vi "UpdateVisibleData.vi"(7 "Templates tree":refnum<vi>, 8 "error in (no error)":errorcluster, 9 "Tag":string, 10 "Keyword":string, 11 "FakedArray in":refnum<class "FakedArray.lvclass">) -> (0 "error out":errorcluster, 3 "FakedArray out":refnum<class "FakedArray.lvclass">)   [LabVIEW 2020, in "FakedArray.lvclass"]
uses:
  FakedArray.lvclass
  FakedArray.lvclass/FakedArray.ctl
  vi.lib/LabVIEW Icon API/lv_icon/Classes/Layer/Layer.lvclass
  vi.lib/LabVIEW Icon API/LabVIEW Icon API.lvlib
  Icon Library/Glyph.lvclass
  vi.lib/LabVIEW Icon API/lv_icon/Controls/Graphic.ctl
panel:
  in  "?":T1
  in  "?":T1[](array[typedef])=[{"Rectangle"={"left"=0, "top"=0, "right"=0, "bottom"=0}, "Path"=path "", "Image"=bytes[0], "Filter"="", "FileName"=""}]
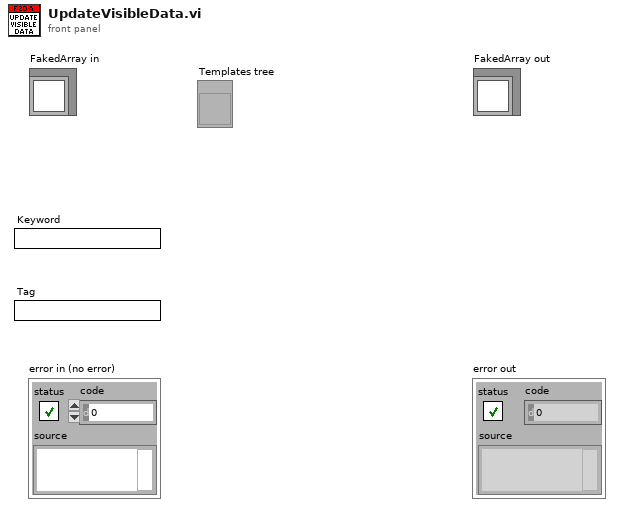
[diagram p1: front panel]
types:
  T1 = typedef "Graphic.ctl" = cluster{"Rectangle":cluster{"left":i16, "top":i16, "right":i16, "bottom":i16}, "Path":path, "Image":picture, "Filter":string, "FileName":string}
  T2 = typedef "ToMoreSpecific_Faked2DArray.ctl" = enum16{"Framework Templates", "Layer List"}
  T3 = typedef "IEColor.ctl" = u32
  T4 = typedef "Path&Icon.ctl" = cluster{"Rectangle":cluster{"left":i16, "top":i16, "right":i16, "bottom":i16}, "Path":path, "Image":picture, "Filter":string, "FileName":string}
  T5 = cluster{"Rectangle":cluster{"left":bool, "top":bool, "right":bool, "bottom":bool}, "Path":bool, "Image":bool, "Filter":bool, "FileName":bool}
  T6 = typedef "Layer.ctl" = cluster{"LayerIcon":picture, "LayerName":string, "Opacity":u8, "Visibility?":bool}
  T7 = typedef "LVPoint32TypeDef.ctl" = cluster{"Horizontal":i32, "Vertical":i32}
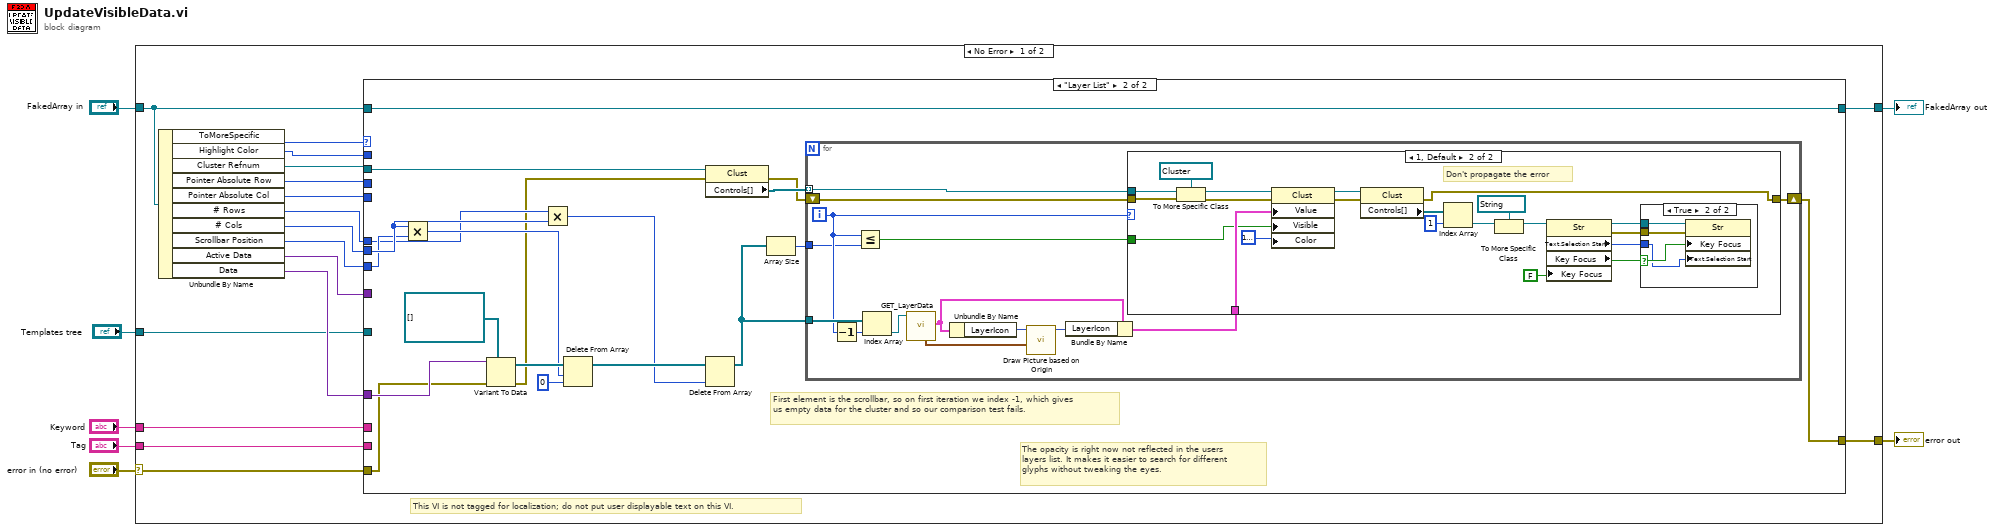
[diagram p0: block diagram]
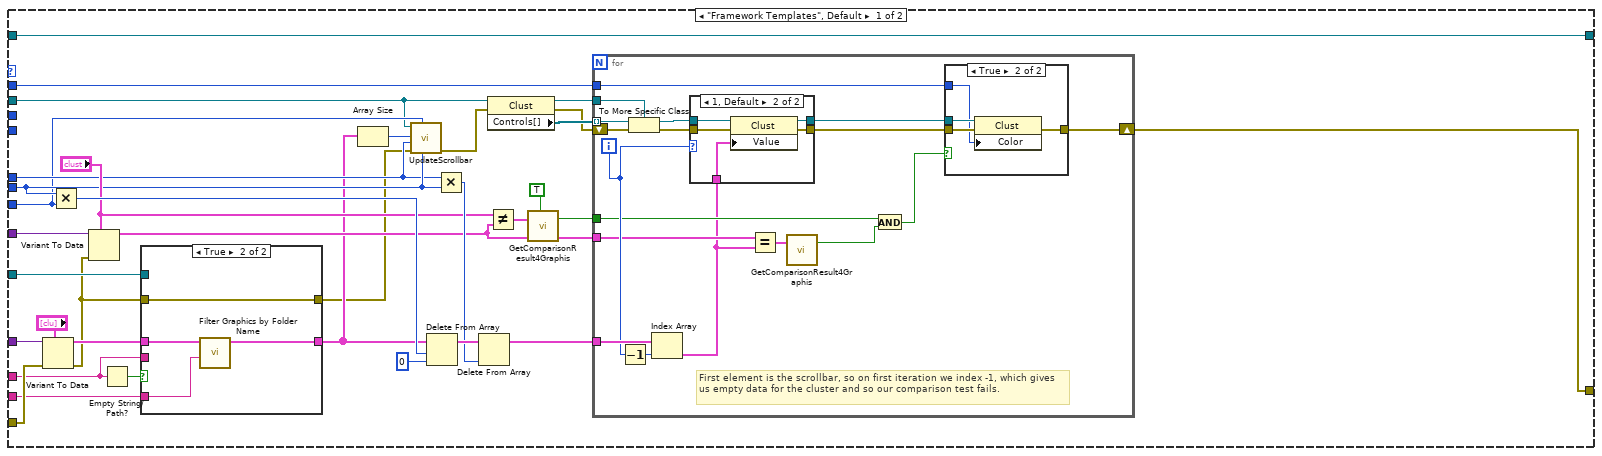
[diagram p2: hidden frame]
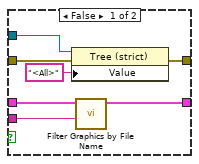
[diagram p3: hidden frame]
diagram:
  n1 = case shown="No Error" "error in (no error)" {
    selector: "error in (no error)" -> [w22 w159]
    tunnel: [w18 w159] -> w6
    tunnel: [w17 w158] -> w4
    tunnel: "FakedArray in" -> [w24 w158]
    tunnel: "Keyword" -> [w14 _]
    tunnel: "Tag" -> [w10 _]
    tunnel: "Templates tree" -> [w8 _]
    frame No Error {
      # "This VI is not tagged for localization; do not put user displayable text on this VI."
      n2 = Unbundle By Name(w24) -> ("ToMoreSpecific"=w9:T2, "Highlight Color"=w11:T3, "Cluster Refnum"=w19:refnum<vi>, "Pointer Absolute Row"=w16:i32, "Pointer Absolute Col"=w15:i32, "# Rows"=w20:i32, "# Cols"=w21:i32, "Scrollbar Position"=w23:i32, "Active Data"=w12:variant, "Data"=w13:variant)
      n3 = case shown="\"Layer List\"" w9 {
        tunnel: w24 -> [w47 w112]
        tunnel: w23 -> [w30 w106]
        tunnel: w13 -> [w58 w117]
        tunnel: w22 -> [w57 w116]
        tunnel: w21 -> [w32 w107]
        tunnel: w20 -> [w31 w102]
        tunnel: w19 -> [w29 w111]
        tunnel: [w48 w113] -> w18
        tunnel: [w47 w112] -> w17
        tunnel: w16 -> [_ _]
        tunnel: w15 -> [_ _]
        tunnel: w14 -> [w43 _]
        tunnel: w12 -> [w42 _]
        tunnel: w11 -> [w37 _]
        tunnel: w10 -> [w35 _]
        tunnel: w8 -> [w34 _]
        frame "Framework Templates", Default {
          n4 = Variant To Data(error in=w57, type="?", Variant=w58) -> (data=w45:T1[], error out=w33:errorcluster)
          n5 = Multiply(x=w32, y=w30) -> (x*y=w55:i32)
          n6 = Variant To Data(error in=w33, type="?", Variant=w42) -> (data=w40:T1)  [unwired: 1 out]
          n7 = Empty String/Path?(string/path=w43) -> (empty?=w44:bool)
          n8 = case shown="True" w44 {
            tunnel: w45 -> [w65 w69]
            tunnel: w43 -> [w64 _]
            tunnel: [w63 w68] -> w28
            tunnel: w35 -> [_ w67]
            tunnel: w33 -> [w60 w66]
            tunnel: [w62 w66] -> w26
            tunnel: w34 -> [w61 _]
            frame False {
              n9 = property class="Tree (strict)"(reference=w61, error in=w60, "Value"="<All>") -> (error out=w62:errorcluster)  [unwired: 1 out]
              n10 = call "Filter Graphics by File Name.vi"("Keyword"=w64, "Icon Templates in"=w65) -> ("Icon Templates out"=w63:T4[])  [unwired: 9 out]
            }
            frame True {
              n11 = call "Filter Graphics by Folder Name.vi"("Tag"=w67, "Glyphs [] in"=w69) -> ("Filtered Glyphs []"=w68:T1[])  [unwired: 9 out]
            }
          }
          n12 = Array Size(array=w28) -> (size(s)=w27:i32)
          n13 = call "UpdateScrollbar.vi"("# Cols"=w32, "Value Scrollbar"=w30, "error in"=w26, "#Rows"=w31, "# Elements"=w27, "Cluster Refnum"=w29) -> ("error out"=w25:errorcluster)  [unwired: 5 out]
          n14 = Delete From Array(array=w28, length=w55, index=0) -> (array with subset deleted=w53:T1[])  [unwired: 1 out]
          n15 = Multiply(x=w31, y=w32) -> (x*y=w52:i32)
          n16 = Delete From Array(array=w53, index=w52) -> (array with subset deleted=w49:T1[])  [unwired: 1 in, 1 out]
          n17 = property class="Clust"(reference=w29, error in=w25) -> (reference out=w46:refnum<vi>, error out=w50:errorcluster, "Controls[]"=w51:refnum<vi>[])
          n18 = Not Equal?(x="?", y=w40) -> (x != y?=w39:T5)
          n19 = call "GetComparisonResult4Graphis.vi"("Comparison In"=w39, "AND vs OR"=TRUE) -> ("True?"=w38:bool)  [unwired: 17 out]
          n20 = for {
            tunnel: w51 -> [w74] mode=indexing
            shift-right: [w76] -> w48
            shift-left: w50 -> [w73]
            tunnel: w49 -> [w87]
            tunnel: w46 -> [w75]
            tunnel: w40 -> [w84]
            tunnel: w38 -> [w82]
            tunnel: w37 -> [w77]
            i -> [w85]
            # "First element is the scrollbar, so on first iteration we index -1, which gives us empty data for the cluster and so our comparison test fails."
            n21 = Decrement(x=w85) -> (x-1=w86:i32)
            n22 = To More Specific Class(target class=w75, reference=w74, error in=w73) -> (specific class reference=w71:refnum<vi>, error out=w72:errorcluster)
            n23 = Index Array(array=w87, index=w86) -> (element=w70:T1)
            n24 = case shown="1, Default" w85 {
              tunnel: w71 -> [w93 w98]
              tunnel: [_ w97] -> w83
              tunnel: w70 -> [_ w96]
              tunnel: [w93 w95] -> w78
              tunnel: w72 -> [_ w94]
              frame 0 {
                # "Do not propagate\nerror! This is the\nscrollbar."
              }
              frame 1, Default {
                n25 = property class="Clust"(reference=w98, error in=w94, "Value"=w96) -> (reference out=w95:refnum<vi>, error out=w97:errorcluster)
              }
            }
            n26 = Equal?(x=w84, y=w70) -> (x = y?=w81:T5)
            n27 = call "GetComparisonResult4Graphis.vi"("Comparison In"=w81) -> ("True?"=w80:bool)  [unwired: 1 in, 17 out]
            n28 = And(x=w82, y=w80) -> (x .and. y?=w79:bool)
            n29 = case shown="True" w79 {
              tunnel: w83 -> [w88 w92]
              tunnel: w78 -> [_ w91]
              tunnel: w77 -> [_ w89]
              tunnel: [w88 w90] -> w76
              frame False {
              }
              frame True {
                n30 = property class="Clust"(reference=w91, error in=w92, "Color"=w89) -> (error out=w90:errorcluster)  [unwired: 1 out]
              }
            }
          }
        }
        frame "Layer List" {
          # "The opacity is right now not reflected in the users\nlayers list. It makes it easier to search for different\nglyphs without tweaking the eyes."
          # "First element is the scrollbar, so on first iteration we index -1, which gives us empty data for the cluster and so our comparison test fails."
          n31 = Multiply(x=w107, y=w106) -> (x*y=w103:i32)
          n32 = Variant To Data(error in=w116, type=refnum<class "Layer.lvclass">[] [] ("All Layers"), Variant=w117) -> (data=w104:refnum<class "Layer.lvclass">[], error out=w99:errorcluster)
          n33 = Multiply(x=w102, y=w107) -> (x*y=w100:i32)
          n34 = Delete From Array(array=w104, length=w103, index=0) -> (array with subset deleted=w108:refnum<class "Layer.lvclass">[])  [unwired: 1 out]
          n35 = property class="Clust"(reference=w111, error in=w99) -> (error out=w114:errorcluster, "Controls[]"=w115:refnum<vi>[])  [unwired: 1 out]
          n36 = Delete From Array(array=w108, index=w100) -> (array with subset deleted=w105:refnum<class "Layer.lvclass">[])  [unwired: 1 in, 1 out]
          n37 = Array Size(array=w105) -> (size(s)=w109:i32)
          n38 = for {
            tunnel: w115 -> [w131] mode=indexing
            shift-right: [w129] -> w113
            shift-left: w114 -> [w130]
            tunnel: w105 -> [w128]
            tunnel: w109 -> [w120]
            i -> [w121]
            n39 = Decrement(x=w121) -> (x-1=w127:i32)
            n40 = Less Or Equal?(x=w121, y=w120) -> (x <= y?=w119:bool)
            n41 = Index Array(array=w128, index=w127) -> (element=w123:refnum<class "Layer.lvclass">)
            n42 = call-dynamic "GET_LayerData.vi"("Layer.lvclass in"=w123) -> ("Data"=w124:T6, "Origin"=w126:T7)  [unwired: 1 in, 8 out]
            n43 = Unbundle By Name(w124) -> ("LayerIcon"=w125:picture)
            n44 = call "Draw Picture based on Origin.vi"("Origin"=w126, "LayerIcon in"=w125) -> ("LayerIcon out"=w118:picture)  [unwired: 1 in, 8 out]
            n45 = Bundle By Name(cluster=w124, "LayerIcon"=w118) -> (w122:T6)
            n46 = case shown="1, Default" w121 {
              tunnel: w131 -> [_ w151]
              tunnel: w130 -> [w132 w150]
              tunnel: [w132 w139] -> w129
              tunnel: w122 -> [_ w153]
              tunnel: w119 -> [_ w152]
              frame 0 {
              }
              frame 1, Default {
                # "Don't propagate the error"
                n47 = To More Specific Class(target class=refnum<vi> refnum ("Cluster Refnum"), reference=w151, error in=w150) -> (specific class reference=w148:refnum<vi>, error out=w147:errorcluster)
                n48 = property class="Clust"(reference=w148, error in=w147, "Value"=w153, "Visible"=w152, "Color"=u32 16777216) -> (reference out=w144:refnum<vi>, error out=w145:errorcluster)
                n49 = property class="Clust"(reference=w144, error in=w145) -> (error out=w139:errorcluster, "Controls[]"=w143:refnum<vi>[])  [unwired: 1 out]
                n50 = Index Array(array=w143, index=1) -> (element=w140:refnum<vi>)
                n51 = To More Specific Class(target class=refnum<vi> refnum ("Cluster Refnum"), reference=w140) -> (specific class reference=w138:refnum<vi>)  [unwired: 1 in, 1 out]
                n52 = property class="Str"(reference=w138, "Key Focus"=FALSE) -> (reference out=w135:refnum<vi>, error out=w134:errorcluster, "Text.Selection Start"=w133:u32, "Key Focus"=w136:bool)  [unwired: 1 in]
                n53 = case shown="True" w136 {
                  selector: w136 -> [_ w155]
                  tunnel: w135 -> [_ w156]
                  tunnel: w134 -> [_ w157]
                  tunnel: w133 -> [_ w154]
                  frame False {
                  }
                  frame True {
                    n54 = property class="Str"(reference=w156, error in=w157, "Key Focus"=w155, "Text.Selection Start"=w154) -> ()  [unwired: 2 out]
                  }
                }
              }
            }
          }
        }
      }
    }
    frame Error {
    }
  }
  "error out" <- w6
  "FakedArray out" <- w4
